vi "Build Decrement Numeric Functions.vi"   [LabVIEW 2021]
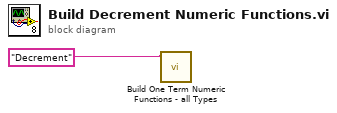
[diagram p0: block diagram]
diagram:
  n1 = call "Build One Term Numeric Functions - all Types.vi"("Comparison Name"="Decrement") -> ()  [unwired: 11 in]
